vi "Done.vi"(8 "error in (no error)":errorcluster, 11 "String Control Sink in":refnum<class "String Control Sink.lvclass">) -> (0 "error out":errorcluster)   [LabVIEW 2019, in "String Control Sink.lvclass"]
doc: "--\nCopyright © 2017 Composed SystemsI All rights reserved.\n\nAuthor: Jon McBee <jon.mcbee@composed.io>\n\nThis library is provided \"AS IS\" ,WITHOUT WARRANTIES OR\nCONDITIONS OF ANY KIND, either express or implied.\n\nComposed Systems -- composed.io\n\nStream 0.0.1.1\nJon McBee - Composed Systems\nCopyright (c) 2017, Composed Systems"
uses:
  String Control Sink.lvclass
  String Control Sink.lvclass/String Control Sink.ctl
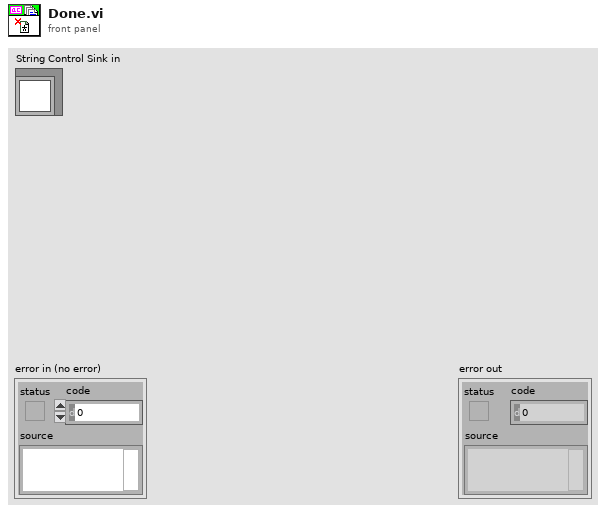
[diagram p1: front panel]
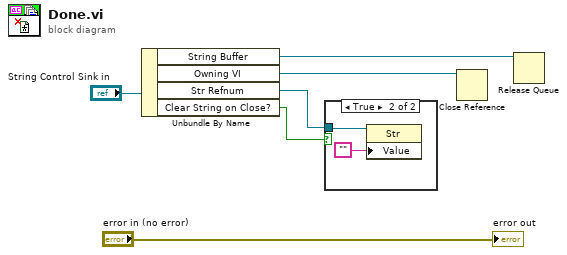
[diagram p0: block diagram]
diagram:
  n1 = Unbundle By Name("String Control Sink in") -> ("String Buffer"=w1:refnum<queue>, "Owning VI"=w4:refnum<vi>, "Str Refnum"=w2:refnum<vi>, "Clear String on Close?"=w3:bool)
  n2 = case shown="True" w3 {
    tunnel: w2 -> [_ w8]
    frame False {
    }
    frame True {
      n3 = property class="Str"(reference=w8, "Value"="") -> ()  [unwired: 1 in, 2 out]
    }
  }
  n4 = Close Reference(reference=w4) -> ()  [unwired: 1 in, 1 out]
  n5 = Release Queue(queue=w1) -> ()  [unwired: 2 in, 3 out]
  "error out" <- "error in (no error)"
